vi "Get Active Buffers.vi"(8 "error in (no error)":errorcluster, 10 "inline?":bool, 11 "Buffers in":refnum<class "Buffers.lvclass">) -> (0 "error out":errorcluster, 1 "engine Buffer":refnum<class "Buffer.lvclass">, 2 "string Buffer":refnum<class "Buffer.lvclass">, 3 "Buffers out":refnum<class "Buffers.lvclass">)   [LabVIEW 2019, in "DSF Core.lvlib" / "Buffers.lvclass"]
uses:
  Buffers.lvclass
  Buffer/Buffer.lvclass
  Buffers.lvclass/Buffers.ctl
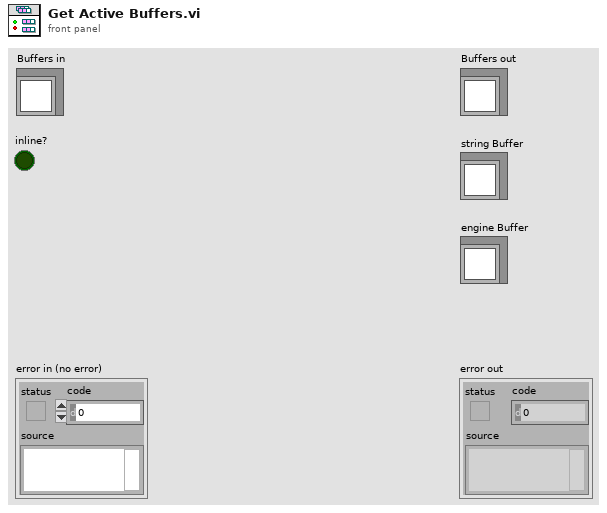
[diagram p1: front panel]
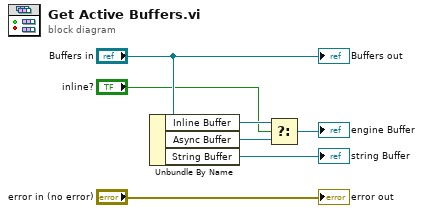
[diagram p0: block diagram]
diagram:
  n1 = Unbundle By Name("Buffers in") -> ("Inline Buffer"=w5:refnum<class "Buffer.lvclass">, "Async Buffer"=w4:refnum<class "Buffer.lvclass">, "String Buffer"=→"string Buffer":refnum<class "Buffer.lvclass">)
  n2 = Select(t=w5, s="inline?", f=w4) -> (s? t:f=→"engine Buffer":refnum<class "Buffer.lvclass">)
  "error out" <- "error in (no error)"
  "Buffers out" <- "Buffers in"
